vi "LS218_READ_8VOIES.vi"(4 "entrée d'erreur (pas d'erreur)":errorcluster, 5 "table_acq_in":T1(array[cluster]), 6 "Celsius":bool, 7 "Refnum VISA en entrée":refnum<visa-resource-name>) -> (0 "sortie d'erreur":errorcluster, 1 "table_acq_out":T1(array[cluster]), 3 "Nom de ressource VISA en sortie":refnum<visa-resource-name>)   [LabVIEW 2016]
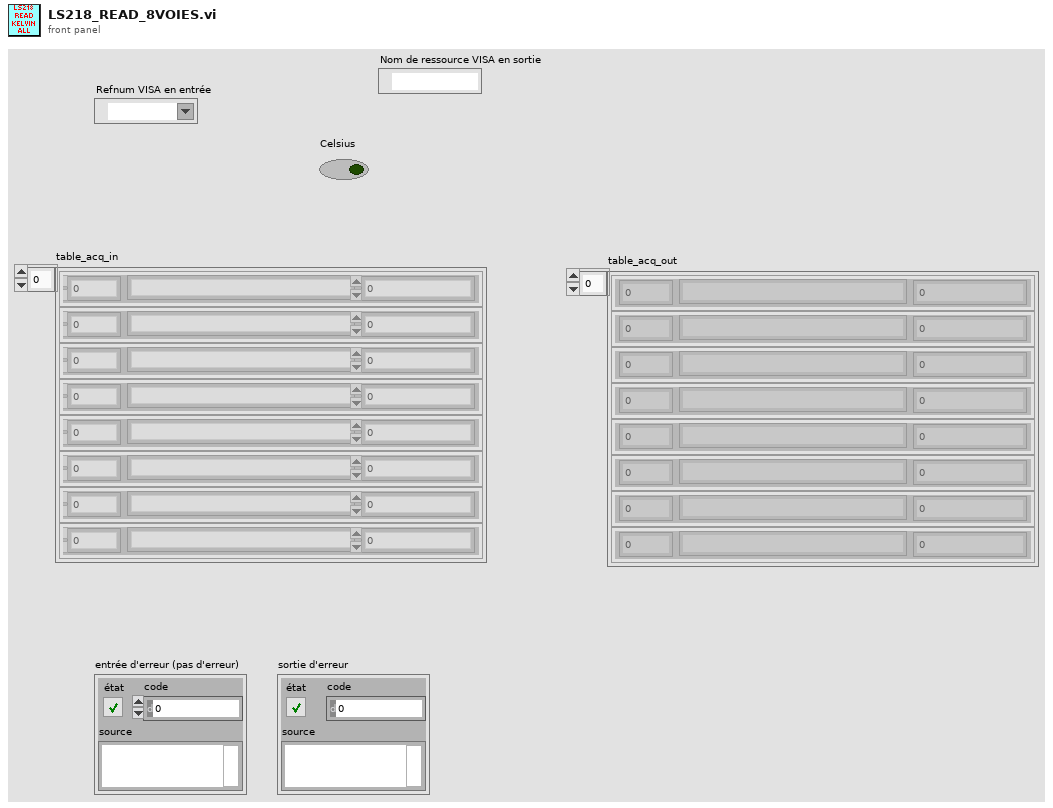
[diagram p1: front panel]
types:
  T1 = cluster{"N_voie":i32, "Nom_voie":string, "Mesure_voie":dbl}[]
  T2 = cluster{"N_voie":i32, "Nom_voie":string, "Mesure_voie":dbl}
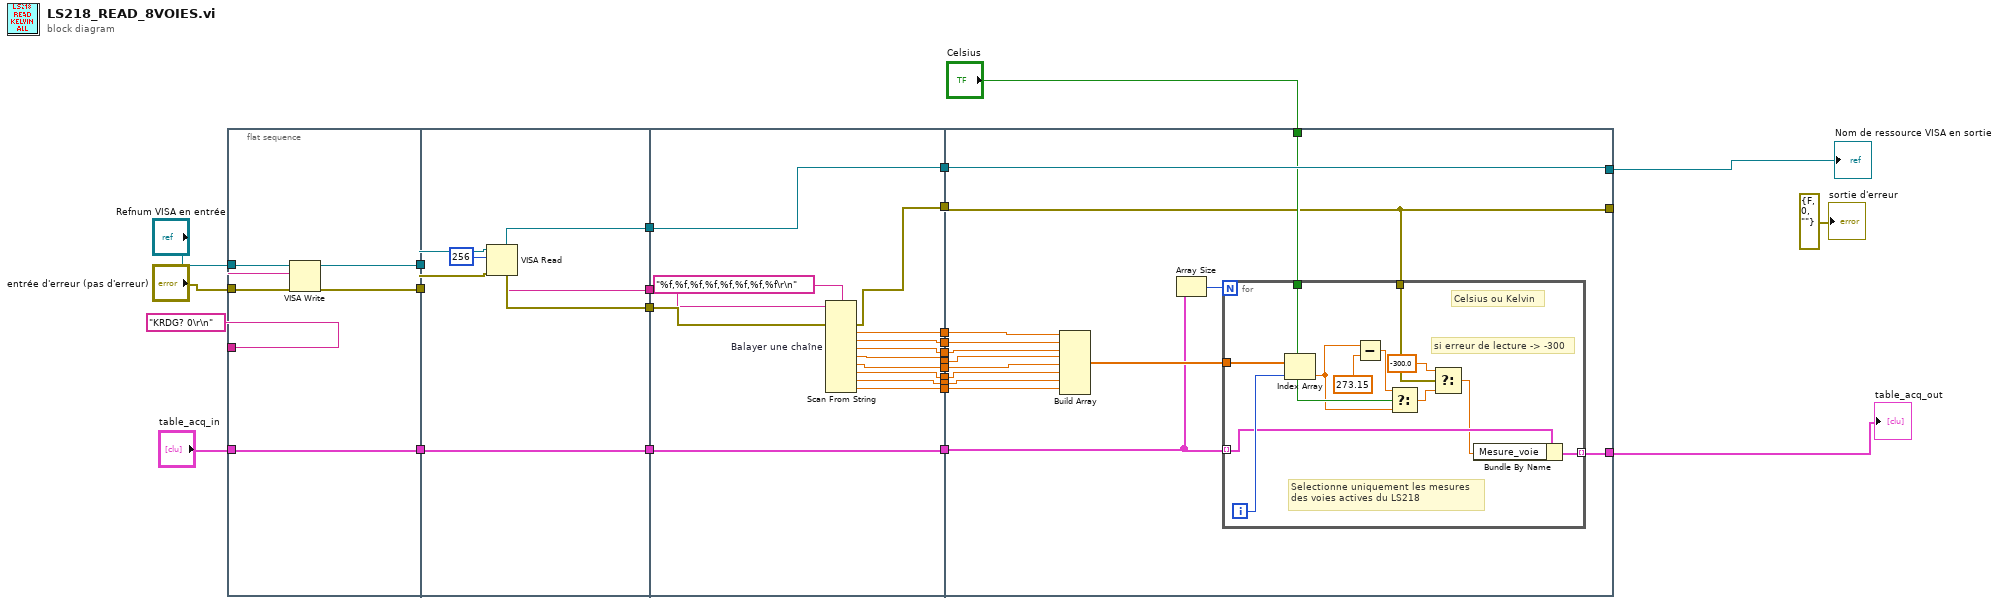
[diagram p0: block diagram]
diagram:
  n1 = flat-sequence {
    tunnel: "Refnum VISA en entrée" -> [w30]
    tunnel: "entrée d'erreur (pas d'erreur)" -> [w29]
    tunnel: "KRDG? 0\r\n" ("chaîne") -> [w28]
    tunnel: [w32] -> w23
    tunnel: [w31] -> w22
    tunnel: [w27] -> w7
    tunnel: "table_acq_in" -> [w27]
    tunnel: w23 -> [w38]
    tunnel: w22 -> [w37]
    tunnel: [w36] -> w20
    tunnel: [w35] -> w19
    tunnel: [w34] -> w18
    tunnel: w7 -> [w33]
    tunnel: [w33] -> w5
    tunnel: w20 -> [w53]
    tunnel: w19 -> [w51]
    tunnel: w18 -> [w50]
    tunnel: [w49] -> w17
    tunnel: [w53] -> w16
    tunnel: [w48] -> w15
    tunnel: [w47] -> w14
    tunnel: [w46] -> w13
    tunnel: [w45] -> w12
    tunnel: [w44] -> w11
    tunnel: [w43] -> w10
    tunnel: [w42] -> w9
    tunnel: [w41] -> w8
    tunnel: w5 -> [w40]
    tunnel: [w40] -> w4
    tunnel: [w68] -> w21
    tunnel: [w54] -> _
    tunnel: w17 -> [w54]
    tunnel: w16 -> [w68]
    tunnel: w15 -> [w67]
    tunnel: w14 -> [w66]
    tunnel: w13 -> [w65]
    tunnel: w12 -> [w64]
    tunnel: w11 -> [w63]
    tunnel: w10 -> [w62]
    tunnel: w9 -> [w61]
    tunnel: w8 -> [w60]
    tunnel: w4 -> [w58]
    tunnel: [w56] -> w3
    tunnel: "Celsius" -> [w55]
    frame #0 {
      n2 = VISA Write(VISA resource name=w30, write buffer=w28, error in (no error)=w29) -> (VISA resource name out=w31:refnum<visa-resource-name>, error out=w32:errorcluster)  [unwired: 1 out]
    }
    frame #1 {
      n3 = VISA Read(VISA resource name=w37, byte count=u32 256 ("nombre d'octets"), error in (no error)=w38) -> (VISA resource name out=w36:refnum<visa-resource-name>, read buffer=w34:string, error out=w35:errorcluster)  [unwired: 1 out]
    }
    frame #2 {
      n4 = Scan From String "Balayer une chaîne"(format string="%f,%f,%f,%f,%f,%f,%f,%f\r\n" ("chaîne de format"), input string=w50, error in=w51) -> (error out=w49:errorcluster, output 1=w48:dbl, output 2=w47:dbl, output 3=w46:dbl, output 4=w45:dbl, output 5=w44:dbl, output 6=w43:dbl, output 7=w42:dbl, output 8=w41:dbl)  [unwired: 9 in, 2 out]
    }
    frame #3 {
      n5 = Build Array(w67, w66, w65, w64, w63, w62, w61, w60) -> (w59:dbl[])
      n6 = Array Size(array=w58) -> (size(s)=w57:i32)
      n7 = for {
        N: w57 -> [_]
        tunnel: w58 -> [w78] mode=indexing
        tunnel: w59 -> [w80]
        tunnel: [w77] -> w56 mode=indexing
        tunnel: w55 -> [w76]
        tunnel: w54 -> [w70]
        i -> [w79]
        # "si erreur de lecture -> -300"
        # "Selectionne uniquement les mesures\ndes voies actives du LS218"
        # "Celsius ou Kelvin"
        n8 = Index Array(array=w80, index=w79) -> (element=w74:dbl)
        n9 = Subtract(x=w74, y=273.15 ("x")) -> (x-y=w75:dbl)
        n10 = Select(t=w75, s=w76, f=w74) -> (s? t:f=w71:dbl)
        n11 = Select(t=-300.0 ("cas vrai"), s=w70, f=w71) -> (s? t:f=w72:dbl)
        n12 = Bundle By Name(cluster=w78, "Mesure_voie"=w72) -> (w77:T2)
      }
    }
  }
  "sortie d'erreur" <- errorcluster {"status"=FALSE, "code"=0, "source"=""} ("sortie d'erreur")
  "Nom de ressource VISA en sortie" <- w21
  "table_acq_out" <- w3
